vi "subop_x2_Acquisition.vi"(0 "ACQ stop by events":T2={"ACQ stop by events button"=FALSE, "Events to acquire"=1000} caption="Stop by events" {"Events to acquire" min=1}, 1 "LayerChipIDs":u16[](array[numeric])=[65535, 65535] format="%04x", 2 "ACQ parameters":u32[](array[numeric])=[0, 0, 0, 0], 3 "events fets A Refnum":refnum<vi>, 4 "events fets B Refnum":refnum<vi>, 5 "Base file path":path=path "C:/VIP Module x2/Files/ACQbinaryData.dat", 6 "Addresses Cluster":T1={"ENA1"=FALSE, "IP address 1"="172.16.14.22", "ENA2"=FALSE, "IP address 2"="172.16.14.23"}, 7 "Stop ACQ button Refnum":refnum<vi>, 8 "ACQ barra Refnum":refnum<vi>, 10 "Actual time Refnum":refnum<vi>, 12 "Acquisition time Refnum":refnum<vi>, 14 "Total events Refnum":refnum<vi>) -> (13 "Stop by events":bool, 15 "ACQ WatchDog timeout":bool, 17 "ACQ Answer 1i2":string, 25 "error out comm":errorcluster, 27 "error out file":errorcluster)   [LabVIEW 2015, in "VIPM2.lvlib"]
uses:
  VIPM2.lvlib
panel:
  out "STOP FPGAs":bool
  out "Ready to receive parameters 2":string
  out "Ready to receive parameters 1":string
  # "Acquisition in progress..."
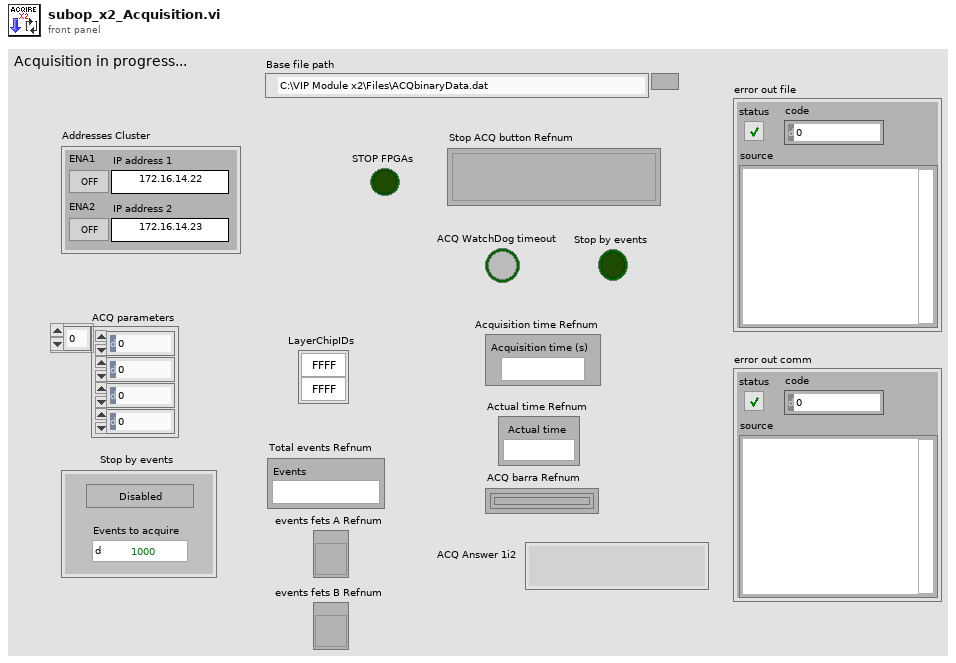
[diagram p1: front panel]
types:
  T1 = cluster{"ENA1":bool, "IP address 1":string, "ENA2":bool, "IP address 2":string}
  T2 = cluster{"ACQ stop by events button":bool, "Events to acquire":u32}
  T3 = enum16{"Standard", "Buffered", "CRLF", "Immediate"}
  T4 = enum16{"open", "replace", "create", "open or create", "replace or create", "replace or create with confirmation"}
  T5 = enum16{"big-endian, network order", "native, host order", "little-endian"}
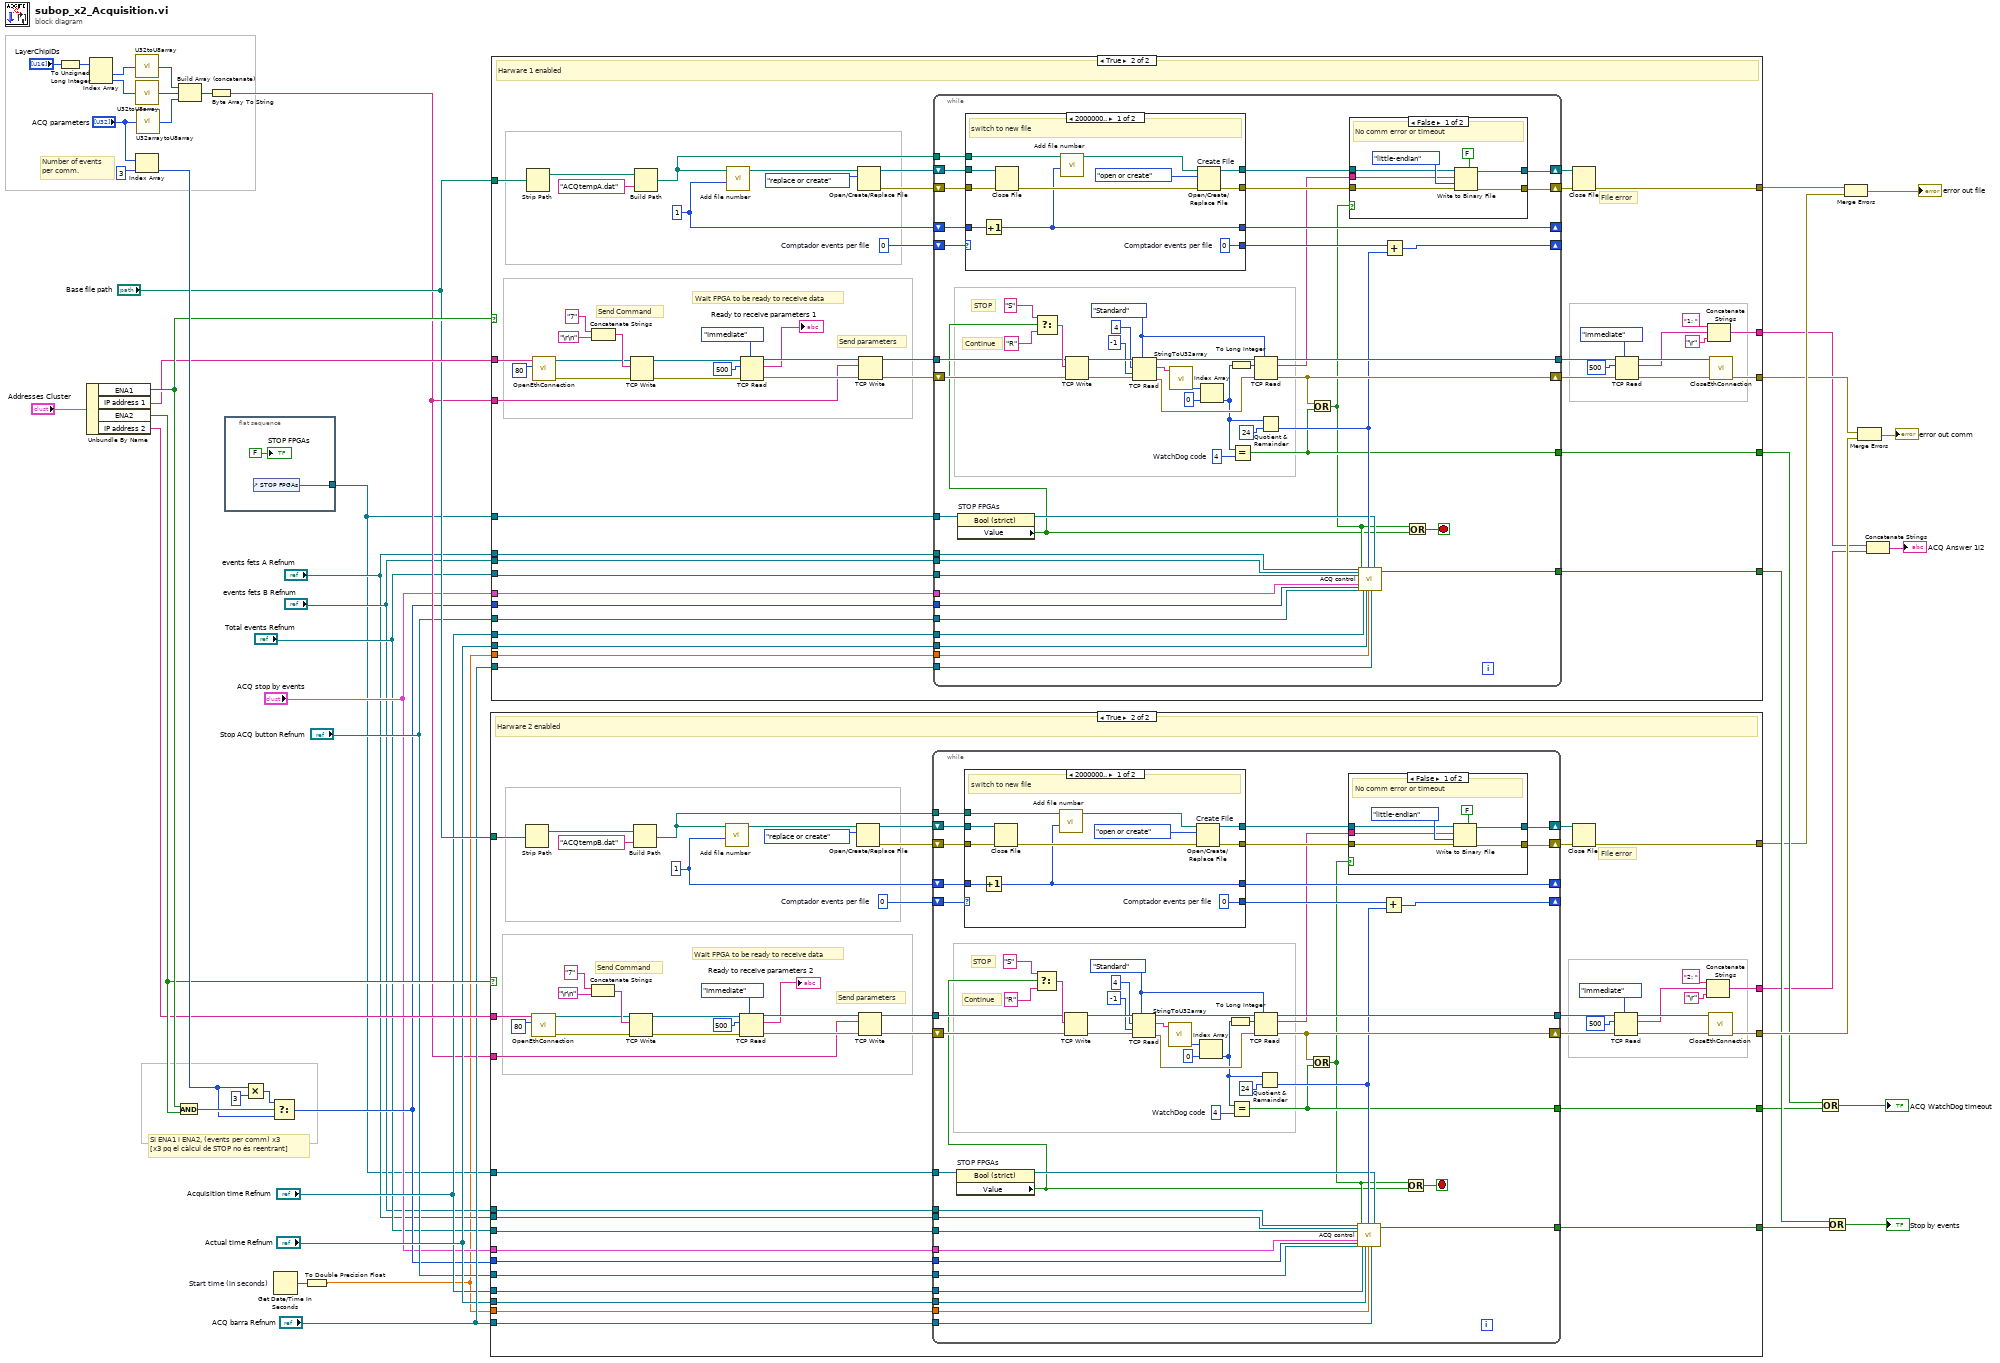
[diagram p0: block diagram]
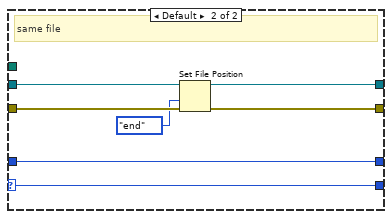
[diagram p3: hidden frame]
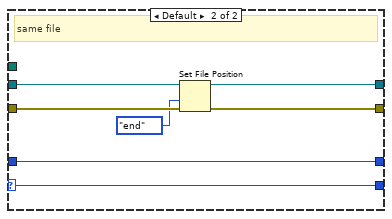
[diagram p6: hidden frame]
diagram:
  # "Si ENA1 i ENA2, (events per comm) x3\n[x3 pq el càlcul de STOP no és reentrant]"
  # "Number of events\nper comm."
  n1 = To Unsigned Long Integer(number="LayerChipIDs") -> (unsigned 32bit integer=w6:u32[])
  n2 = Unbundle By Name("Addresses Cluster") -> ("ENA1"=w35:bool, "IP address 1"=w34:string, "ENA2"=w32:bool, "IP address 2"=w31:string)
  n3 = Index Array "Index Array"(array=w6) -> (element #1=w4:u32, element #2=w3:u32)  [unwired: 2 in]
  n4 = call "U32toU8array.vi"("x"=w4) -> ("ArrayU8"=w41:u8[])
  n5 = call "U32toU8array.vi"("x"=w3) -> ("ArrayU8"=w5:u8[])
  n6 = Index Array "Index Array"(array="ACQ parameters", index=3) -> (element=w37:u32)
  n7 = call "U32arraytoU8array.vi"("ArrayU32"="ACQ parameters") -> ("ArrayU8"=w46:u8[])
  n8 = And(x=w35, y=w32) -> (x .and. y?=w40:bool)
  n9 = Build Array (concatenate)(w41, w5, w46) -> (w47:u8[])
  n10 = Byte Array To String(unsigned byte array=w47) -> (string=w27:string)
  n11 = flat-sequence {
    tunnel: [w49] -> w20
    frame #0 {
      n12 = control-ref of="STOP FPGAs"() -> (w49:refnum<vi>)
      "STOP FPGAs" <- FALSE ("STOP FPGAs")
    }
  }
  n13 = Multiply(x=w37, y=u32 3) -> (x*y=w39:u32)
  n14 = Select(t=w39, s=w40, f=w37) -> (s? t:f=w25:u32)
  n15 = Get Date/Time In Seconds "Start time (in seconds)"() -> (seconds since 1Jan1904=w2:timestamp)
  n16 = To Double Precision Float(number=w2) -> (double precision float=w1:dbl)
  n17 = case shown="True" w32 {
    tunnel: "Base file path" -> [_ w70]
    tunnel: w31 -> [_ w69]
    tunnel: w27 -> [_ w68]
    tunnel: "ACQ stop by events" -> [_ w67]
    tunnel: w25 -> [_ w66]
    tunnel: "Stop ACQ button Refnum" -> [_ w65]
    tunnel: "Acquisition time Refnum" -> [_ w64]
    tunnel: "Actual time Refnum" -> [_ w63]
    tunnel: w1 -> [_ w62]
    tunnel: "ACQ barra Refnum" -> [_ w61]
    tunnel: [_ w60] -> w19
    tunnel: [_ w59] -> w12
    tunnel: [_ w58] -> w8
    tunnel: [_ w57] -> w48
    tunnel: "events fets B Refnum" -> [_ w56]
    tunnel: "events fets A Refnum" -> [_ w55]
    tunnel: "Total events Refnum" -> [_ w54]
    tunnel: w20 -> [_ w53]
    tunnel: [_ w52] -> w16
    frame False {
      # "Hardware 1 not enabled"
    }
    frame True {
      w84 = u32 0  # Comptador events per file
      w85 = u32 1 ("sufix number")
      # "File error"
      # "Send parameters"
      # "Wait FPGA to be ready to receive data"
      # "Send Command"
      # "Harware 2 enabled"
      n18 = Strip Path(path=w70) -> (stripped path=w92:path)  [unwired: 1 out]
      n19 = call "OpenEthConnection.vi"("Port"=u16 80, "IP address"=w69) -> ("error out"=w94:errorcluster, "connection ID out"=w95:refnum<k5>)  [unwired: 7 in, 1 out]
      n20 = Concatenate Strings("7" ("string"), "\r\n") -> (w102:string)
      n21 = TCP Write(connection ID=w95, data in=w102, error in (no error)=w94) -> (connection ID out=w99:refnum<k5>, error out=w98:errorcluster)  [unwired: 1 in, 1 out]
      n22 = Build Path(base path=w92, name or relative path="ACQtempB.dat") -> (appended path=w88:path)
      n23 = call "Add file number.vi"("sufix number"=w85, "file path"=w88) -> ("incremented file path"=w90:path)  [unwired: 9 in]
      n24 = TCP Read(connection ID=w99, bytes to read=500, error in (no error)=w98, 7:T3."Immediate" ("mode (standard)")) -> (connection ID out=w97:refnum<k5>, data out=→"Ready to receive parameters 2":string, error out=w96:errorcluster)  [unwired: 1 in]
      n25 = Open/Create/Replace File(file path (use dialog)=w90, operation (0:open)=T4."replace or create") -> (refnum out=w87:refnum<file>, error out=w86:errorcluster)  [unwired: 4 in, 1 out]
      n26 = TCP Write(connection ID=w97, data in=w68, error in (no error)=w96) -> (connection ID out=w83:refnum<k5>, error out=w82:errorcluster)  [unwired: 1 in, 1 out]
      n27 = while {
        tunnel: w88 -> [w139]
        tunnel: w83 -> [w134]
        shift-right: [w131] -> w81
        shift-left: w87 -> [w138]
        shift-right: [w129] -> w80
        shift-left: w86 -> [w137]
        shift-right: [w127] -> _
        shift-left: w85 -> [w136]
        shift-right: [w125] -> _
        shift-left: w84 -> [w135]
        shift-right: [w123] -> w71
        shift-left: w82 -> [w133]
        tunnel: [w128] -> w72
        tunnel: w65 -> [w117]
        tunnel: w67 -> [w119]
        tunnel: w66 -> [w118]
        tunnel: w64 -> [w116]
        tunnel: w63 -> [w115]
        tunnel: w62 -> [w114]
        tunnel: w61 -> [w113]
        tunnel: [w112] -> w60
        tunnel: w56 -> [w122]
        tunnel: w55 -> [w121]
        tunnel: w54 -> [w120]
        tunnel: w53 -> [w110]
        tunnel: [w108] -> w52
        stop <- w105 stop-if-true
        w149 = u32 4  # WatchDog code
        w152 = T3."Standard" ("mode (standard)")
        # "Continue"
        # "STOP"
        n28 = property on="STOP FPGAs" class="Bool (strict)"(reference=w110) -> (reference out=w109:refnum<vi>, "Value"=w106:bool)  [unwired: 1 in, 1 out]
        n29 = case shown="2000000.." w135 {
          selector: w135 -> [_ w169]
          tunnel: w138 -> [w165 w174]
          tunnel: w137 -> [w166 w173]
          tunnel: [w159 w171] -> w130
          tunnel: [w160 w170] -> w132
          tunnel: [w167 w169] -> w126
          tunnel: [w157 w168] -> w127
          tunnel: w136 -> [w164 w168]
          tunnel: w139 -> [w163 _]
          frame 2000000.. {
            w167 = u32 0  # Comptador events per file
            # "switch to new file"
            n30 = Increment(x=w164) -> (x+1=w157:u32)
            n31 = Close File(refnum=w165, error in=w166) -> (error out=w158:errorcluster)  [unwired: 1 out]
            n32 = call "Add file number.vi"("sufix number"=w157, "file path"=w163) -> ("incremented file path"=w162:path)  [unwired: 9 in]
            n33 = Open/Create/Replace File "Create File"(file path (use dialog)=w162, error in=w158, operation (0:open)=T4."open or create") -> (refnum out=w160:refnum<file>, error out=w159:errorcluster)  [unwired: 3 in, 1 out]
          }
          frame Default {
            # "same file"
            n34 = Set File Position(refnum=w174, from (0:start)=enum16{"start", "end", "current"}."end", error in=w173) -> (refnum out=w170:refnum<file>, error out=w171:errorcluster)  [unwired: 1 in]
          }
        }
        n35 = Select(t="S" ("string"), s=w106, f="R" ("string")) -> (s? t:f=w154:string)
        n36 = TCP Write(connection ID=w134, data in=w154, error in (no error)=w133) -> (connection ID out=w148:refnum<k5>, error out=w147:errorcluster)  [unwired: 1 in, 1 out]
        n37 = TCP Read(connection ID=w148, bytes to read=4, error in (no error)=w147, 7:w152, 9:-1 ("timeout ms (25000)")) -> (connection ID out=w150:refnum<k5>, data out=w146:string, error out=w151:errorcluster)
        n38 = call "StringToU32array.vi"("String"=w146) -> ("U32array"=w145:u32[])  [unwired: 2 out]
        n39 = Index Array(array=w145, index=0) -> (element=w142:u32)
        n40 = To Long Integer(number=w142) -> (32bit integer=w143:i32)
        n41 = Equal?(x=w142, y=w149) -> (x = y?=w108:bool)
        n42 = TCP Read(connection ID=w150, bytes to read=w143, error in (no error)=w151, 7:w152) -> (connection ID out=w128:refnum<k5>, data out=w124:string, error out=w123:errorcluster)  [unwired: 1 in]
        n43 = Quotient & Remainder(x=w142, y=u32 24) -> (floor(x/y)=w111:u32)  [unwired: 1 out]
        n44 = Or(x=w123, y=w108) -> (x .or. y?=w107:bool)
        n45 = case shown="False" w107 {
          tunnel: [w179 w183] -> w131
          tunnel: [w178 w182] -> w129
          tunnel: w124 -> [w177 _]
          tunnel: w130 -> [w176 w182]
          tunnel: w132 -> [w175 w183]
          frame False {
            # "No comm error or timeout"
            n46 = Write to Binary File(file (use dialog)=w175, data=w177, error in=w176, 5:FALSE ("prepend array or string size? (T)"), 9:T5."little-endian" ("byte order (0:big-endian, network order)")) -> (refnum out=w179:refnum<file>, error out=w178:errorcluster)  [unwired: 1 in, 1 out]
          }
          frame True {
          }
        }
        n47 = call "ACQ control.vi"("events fets propi Refnum"=w122, "events fets altre Refnum"=w121, "Total events Refnum"=w120, "ACQ stop by events"=w119, "events per comm"=w118, "Stop ACQ button Refnum"=w117, "comm error or timeout"=w107, "Acquisition time Refnum"=w116, "Actual time Refnum"=w115, "events propi"=w111, "start time (in seconds)"=w114, "ACQ barra Refnum"=w113, "STOP FPGAs Refnum"=w109) -> ("Stop by events"=w112:bool)  [unwired: 14 in]
        n48 = Add(x=w126, y=w111) -> (x+y=w125:u32)
        n49 = Or(x=w107, y=w106) -> (x .or. y?=w105:bool)
      }
      n50 = Close File(refnum=w81, error in=w80) -> (error out=w59:errorcluster)  [unwired: 1 out]
      n51 = TCP Read(connection ID=w72, bytes to read=500, error in (no error)=w71, 7:T3."Immediate" ("mode (standard)")) -> (connection ID out=w77:refnum<k5>, data out=w74:string, error out=w76:errorcluster)  [unwired: 1 in]
      n52 = Concatenate Strings("2: " ("string"), w74, "\r") -> (w58:string)
      n53 = call "CloseEthConnection.vi"("error in (no error)"=w76, "connection ID"=w77) -> ("error out"=w57:errorcluster)  [unwired: 9 in]
    }
  }
  n54 = case shown="True" w35 {
    tunnel: "Base file path" -> [_ w203]
    tunnel: w34 -> [_ w202]
    tunnel: w27 -> [_ w201]
    tunnel: "ACQ stop by events" -> [_ w200]
    tunnel: w25 -> [_ w199]
    tunnel: "Stop ACQ button Refnum" -> [_ w198]
    tunnel: "Acquisition time Refnum" -> [_ w197]
    tunnel: "Actual time Refnum" -> [_ w196]
    tunnel: w1 -> [_ w195]
    tunnel: "ACQ barra Refnum" -> [_ w194]
    tunnel: [_ w193] -> w18
    tunnel: [_ w192] -> w13
    tunnel: [_ w191] -> w9
    tunnel: [_ w190] -> w10
    tunnel: "events fets A Refnum" -> [_ w189]
    tunnel: "events fets B Refnum" -> [_ w188]
    tunnel: "Total events Refnum" -> [_ w187]
    tunnel: w20 -> [_ w186]
    tunnel: [_ w185] -> w15
    frame False {
      # "Hardware 1 not enabled"
    }
    frame True {
      w217 = u32 0  # Comptador events per file
      w218 = u32 1 ("sufix number")
      # "File error"
      # "Send parameters"
      # "Wait FPGA to be ready to receive data"
      # "Send Command"
      # "Harware 1 enabled"
      n55 = Strip Path(path=w203) -> (stripped path=w225:path)  [unwired: 1 out]
      n56 = call "OpenEthConnection.vi"("Port"=u16 80, "IP address"=w202) -> ("error out"=w227:errorcluster, "connection ID out"=w228:refnum<k5>)  [unwired: 7 in, 1 out]
      n57 = Concatenate Strings("7" ("string"), "\r\n") -> (w235:string)
      n58 = TCP Write(connection ID=w228, data in=w235, error in (no error)=w227) -> (connection ID out=w232:refnum<k5>, error out=w231:errorcluster)  [unwired: 1 in, 1 out]
      n59 = Build Path(base path=w225, name or relative path="ACQtempA.dat") -> (appended path=w221:path)
      n60 = call "Add file number.vi"("sufix number"=w218, "file path"=w221) -> ("incremented file path"=w223:path)  [unwired: 9 in]
      n61 = TCP Read(connection ID=w232, bytes to read=500, error in (no error)=w231, 7:T3."Immediate" ("mode (standard)")) -> (connection ID out=w230:refnum<k5>, data out=→"Ready to receive parameters 1":string, error out=w229:errorcluster)  [unwired: 1 in]
      n62 = Open/Create/Replace File(file path (use dialog)=w223, operation (0:open)=T4."replace or create") -> (refnum out=w220:refnum<file>, error out=w219:errorcluster)  [unwired: 4 in, 1 out]
      n63 = TCP Write(connection ID=w230, data in=w201, error in (no error)=w229) -> (connection ID out=w216:refnum<k5>, error out=w215:errorcluster)  [unwired: 1 in, 1 out]
      n64 = while {
        tunnel: w221 -> [w272]
        tunnel: w216 -> [w267]
        shift-right: [w264] -> w214
        shift-left: w220 -> [w271]
        shift-right: [w262] -> w213
        shift-left: w219 -> [w270]
        shift-right: [w260] -> _
        shift-left: w218 -> [w269]
        shift-right: [w258] -> _
        shift-left: w217 -> [w268]
        shift-right: [w256] -> w204
        shift-left: w215 -> [w266]
        tunnel: [w261] -> w205
        tunnel: w198 -> [w250]
        tunnel: w200 -> [w252]
        tunnel: w199 -> [w251]
        tunnel: w197 -> [w249]
        tunnel: w196 -> [w248]
        tunnel: w195 -> [w247]
        tunnel: w194 -> [w246]
        tunnel: [w245] -> w193
        tunnel: w189 -> [w255]
        tunnel: w188 -> [w254]
        tunnel: w187 -> [w253]
        tunnel: w186 -> [w243]
        tunnel: [w241] -> w185
        stop <- w238 stop-if-true
        w282 = u32 4  # WatchDog code
        w285 = T3."Standard" ("mode (standard)")
        # "Continue"
        # "STOP"
        n65 = property on="STOP FPGAs" class="Bool (strict)"(reference=w243) -> (reference out=w242:refnum<vi>, "Value"=w239:bool)  [unwired: 1 in, 1 out]
        n66 = case shown="2000000.." w268 {
          selector: w268 -> [_ w302]
          tunnel: w271 -> [w298 w307]
          tunnel: w270 -> [w299 w306]
          tunnel: [w292 w304] -> w263
          tunnel: [w293 w303] -> w265
          tunnel: [w300 w302] -> w259
          tunnel: [w290 w301] -> w260
          tunnel: w269 -> [w297 w301]
          tunnel: w272 -> [w296 _]
          frame 2000000.. {
            w300 = u32 0  # Comptador events per file
            # "switch to new file"
            n67 = Increment(x=w297) -> (x+1=w290:u32)
            n68 = Close File(refnum=w298, error in=w299) -> (error out=w291:errorcluster)  [unwired: 1 out]
            n69 = call "Add file number.vi"("sufix number"=w290, "file path"=w296) -> ("incremented file path"=w295:path)  [unwired: 9 in]
            n70 = Open/Create/Replace File "Create File"(file path (use dialog)=w295, error in=w291, operation (0:open)=T4."open or create") -> (refnum out=w293:refnum<file>, error out=w292:errorcluster)  [unwired: 3 in, 1 out]
          }
          frame Default {
            # "same file"
            n71 = Set File Position(refnum=w307, from (0:start)=enum16{"start", "end", "current"}."end", error in=w306) -> (refnum out=w303:refnum<file>, error out=w304:errorcluster)  [unwired: 1 in]
          }
        }
        n72 = Select(t="S" ("string"), s=w239, f="R" ("string")) -> (s? t:f=w287:string)
        n73 = TCP Write(connection ID=w267, data in=w287, error in (no error)=w266) -> (connection ID out=w281:refnum<k5>, error out=w280:errorcluster)  [unwired: 1 in, 1 out]
        n74 = TCP Read(connection ID=w281, bytes to read=4, error in (no error)=w280, 7:w285, 9:-1 ("timeout ms (25000)")) -> (connection ID out=w283:refnum<k5>, data out=w279:string, error out=w284:errorcluster)
        n75 = call "StringToU32array.vi"("String"=w279) -> ("U32array"=w278:u32[])  [unwired: 2 out]
        n76 = Index Array(array=w278, index=0) -> (element=w275:u32)
        n77 = To Long Integer(number=w275) -> (32bit integer=w276:i32)
        n78 = Equal?(x=w275, y=w282) -> (x = y?=w241:bool)
        n79 = TCP Read(connection ID=w283, bytes to read=w276, error in (no error)=w284, 7:w285) -> (connection ID out=w261:refnum<k5>, data out=w257:string, error out=w256:errorcluster)  [unwired: 1 in]
        n80 = Quotient & Remainder(x=w275, y=u32 24) -> (floor(x/y)=w244:u32)  [unwired: 1 out]
        n81 = Or(x=w256, y=w241) -> (x .or. y?=w240:bool)
        n82 = case shown="False" w240 {
          tunnel: [w312 w316] -> w264
          tunnel: [w311 w315] -> w262
          tunnel: w257 -> [w310 _]
          tunnel: w263 -> [w309 w315]
          tunnel: w265 -> [w308 w316]
          frame False {
            # "No comm error or timeout"
            n83 = Write to Binary File(file (use dialog)=w308, data=w310, error in=w309, 5:FALSE ("prepend array or string size? (T)"), 9:T5."little-endian" ("byte order (0:big-endian, network order)")) -> (refnum out=w312:refnum<file>, error out=w311:errorcluster)  [unwired: 1 in, 1 out]
          }
          frame True {
          }
        }
        n84 = call "ACQ control.vi"("events fets propi Refnum"=w255, "events fets altre Refnum"=w254, "Total events Refnum"=w253, "ACQ stop by events"=w252, "events per comm"=w251, "Stop ACQ button Refnum"=w250, "comm error or timeout"=w240, "Acquisition time Refnum"=w249, "Actual time Refnum"=w248, "events propi"=w244, "start time (in seconds)"=w247, "ACQ barra Refnum"=w246, "STOP FPGAs Refnum"=w242) -> ("Stop by events"=w245:bool)  [unwired: 14 in]
        n85 = Add(x=w259, y=w244) -> (x+y=w258:u32)
        n86 = Or(x=w240, y=w239) -> (x .or. y?=w238:bool)
      }
      n87 = Close File(refnum=w214, error in=w213) -> (error out=w192:errorcluster)  [unwired: 1 out]
      n88 = TCP Read(connection ID=w205, bytes to read=500, error in (no error)=w204, 7:T3."Immediate" ("mode (standard)")) -> (connection ID out=w210:refnum<k5>, data out=w207:string, error out=w209:errorcluster)  [unwired: 1 in]
      n89 = Concatenate Strings("1: " ("string"), w207, "\r") -> (w191:string)
      n90 = call "CloseEthConnection.vi"("error in (no error)"=w209, "connection ID"=w210) -> ("error out"=w190:errorcluster)  [unwired: 9 in]
    }
  }
  n91 = Or(x=w15, y=w16) -> (x .or. y?=→"ACQ WatchDog timeout":bool)
  n92 = Or(x=w18, y=w19) -> (x .or. y?=→"Stop by events":bool)
  n93 = Merge Errors "Merge Errors"(w13, w12) -> (→"error out file":errorcluster)
  n94 = Merge Errors "Merge Errors"(w10, w48) -> (→"error out comm":errorcluster)
  n95 = Concatenate Strings "Concatenate Strings"(w9, w8) -> (→"ACQ Answer 1i2":string)
